vi "MeasureRMS.vi"(8 "# of Samples":dbl, 11 "Sampling Rate (Hz)":dbl) -> (0 "Waveform Graph":dynamicdata(graph), 3 "RMS":dbl)   [LabVIEW 2014]
uses:
  <vilib>/Analysis/5stat.llb/RMS (DBL).vi
  <vilib>/Analysis/NI_AALPro.lvlib
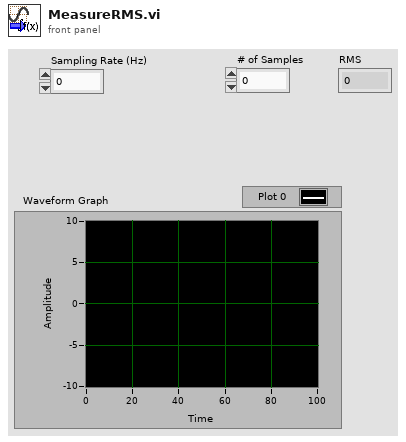
[diagram p1: front panel]
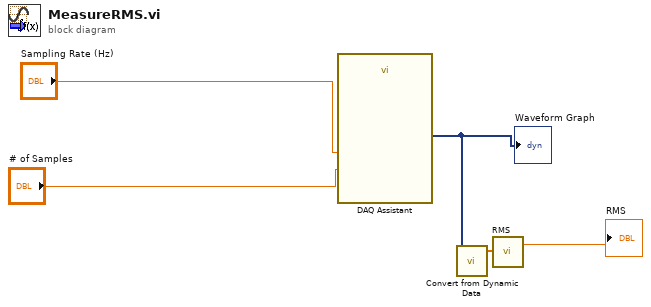
[diagram p0: block diagram]
diagram:
  n1 = call "DAQ Assistant"("rate"="Sampling Rate (Hz)", "number of samples"="# of Samples") -> ("data"=w3:dynamicdata)  [unwired: 15 in, 2 out]
  "Waveform Graph" <- w3
  n2 = call "Convert from Dynamic Data"("Dynamic Data Type"=w3) -> ("Array"=w2:dbl[])  [unwired: 3 in]
  n3 = call-poly <vilib>:"RMS.vi"("X"=w2) -> ("rms value"=→"RMS":dbl)  [unwired: 1 out]
